vi "AlliGator Rescale 2-Exp Fraction.vi"(9 "2-Exp Parameters":T1, 11 "a 1 in":dbl) -> (3 "r 1 out":dbl)   [LabVIEW 2021, in "AlliGator Fit Method Benchmark.lvlib"]
doc: "Normalizes decay amplitudes for random timestamp generation."
uses:
  AlliGator Fit Method Benchmark.lvlib
  AlliGator 2-Exp Parameters.ctl
panel:
  # "see the AlliGator License on the block diagram (Ctrl+E or Window:Show Block Diagram)"
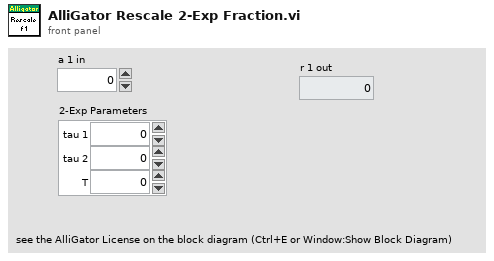
[diagram p1: front panel]
types:
  T1 = typedef "AlliGator Fit Method Benchmark.lvlib/AlliGator 2-Exp Parameters.ctl" = cluster{"tau 1":dbl, "tau 2":dbl, "T":dbl}
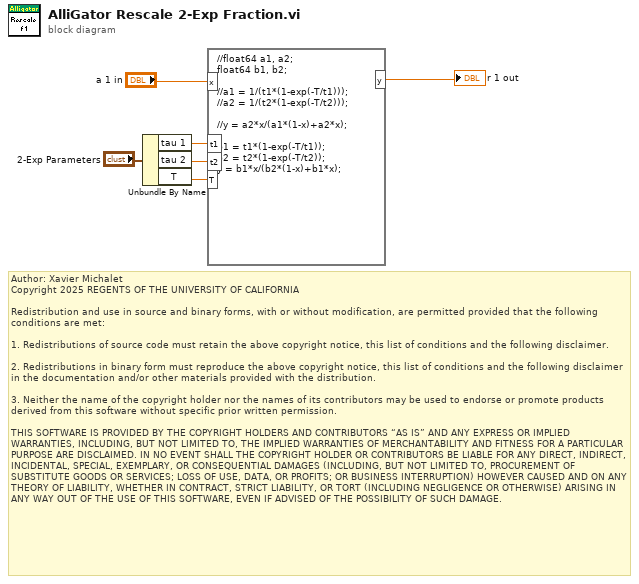
[diagram p0: block diagram]
diagram:
  # "Author: Xavier Michalet\nCopyright 2025 REGENTS OF THE UNIVERSITY OF CALIFORNIA\n\nRedistribution and use in source and binary forms, with or without modification, are permitted provided that the following conditions are met:\n\n1. Redistributions of source code must retain the above copyright notice, this list of conditions and the following disclaimer.\n\n2. Redistributions in binary form must reproduce the above copyright notice, this list of conditions and the following disclaimer in the documentation and/or other materials provided with the distribution.\n\n3. Neither the name of the copyright holder nor the names of its contributors may be used to endorse or promote products derived from this software without specific prior written permission.\n\nTHIS SOFTWARE IS PROVIDED BY THE COPYRIGHT HOLDERS AND CONTRIBUTORS “AS IS” AND ANY EXPRESS OR IMPLIED WARRANTIES, INCLUDING, BUT NOT LIMITED TO, THE IMPLIED WARRANTIES OF MERCHANTABILITY AND FITNESS FOR A PARTICULAR PURPOSE ARE DISCLAIMED. IN NO EVENT SHALL THE COPYRIGHT HOLDER OR CONTRIBUTORS BE LIABLE FOR ANY DIRECT, INDIRECT, INCIDENTAL, SPECIAL, EXEMPLARY, OR CONSEQUENTIAL DAMAGES (INCLUDING, BUT NOT LIMITED TO, PROCUREMENT OF SUBSTITUTE GOODS OR SERVICES; LOSS OF USE, DATA, OR PROFITS; OR BUSINESS INTERRUPTION) HOWEVER CAUSED AND ON ANY THEORY OF LIABILITY, WHETHER IN CONTRACT, STRICT LIABILITY, OR TORT (INCLUDING NEGLIGENCE OR OTHERWISE) ARISING IN ANY WAY OUT OF THE USE OF THIS SOFTWARE, EVEN IF ADVISED OF THE POSSIBILITY OF SUCH DAMAGE."
  n1 = Unbundle By Name("2-Exp Parameters") -> ("tau 1"=w3:dbl, "tau 2"=w2:dbl, "T"=w1:dbl)
  n2 = formula code="//float64 a1, a2;\nfloat64 b1, b2;\n\n//a1 = 1/(t1*(1-exp(-T/t1)));\n//a2 = 1/(t2*(1-exp(-T/t2)));\n\n//y = a2*x/(a1*(1-x)+a2*x);\n\nb1 = t1*(1-exp(-T/t1));\nb2 = t2*(1-exp(-T/t2));\ny = b1*x/(b2*(1-x)+b1*x);"("x"="a 1 in", "t1"=w3, "t2"=w2, "T"=w1) -> ("y"=→"r 1 out":dbl)
